vi "read_attributes.vi"(8 "error in (no error)":errorcluster, 11 "Ridge in":refnum<class "Ridge.lvclass">) -> (0 "error out":errorcluster, 2 "attributes":T1, 3 "Ridge out":refnum<class "Ridge.lvclass">)   [LabVIEW 2020, in "Ridge.lvclass"]
uses:
  Ridge.lvclass
  Controls/ridge_attributes.ctl
  Ridge.lvclass/Ridge.ctl
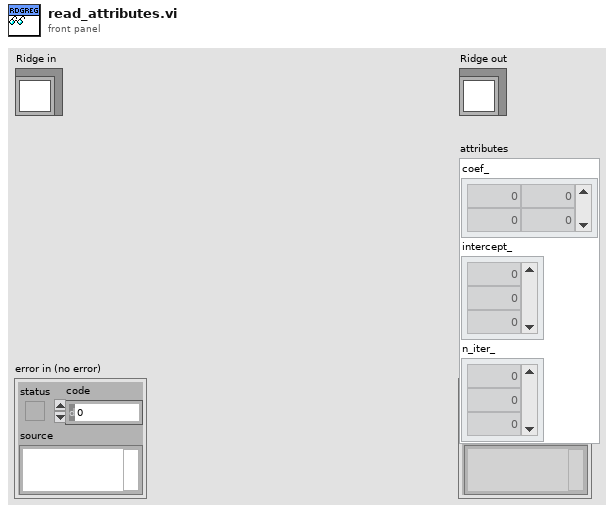
[diagram p1: front panel]
types:
  T1 = typedef "ridge_attributes.ctl" = cluster{"coef_":dbl[][], "intercept_":dbl[], "n_iter_":dbl[]}
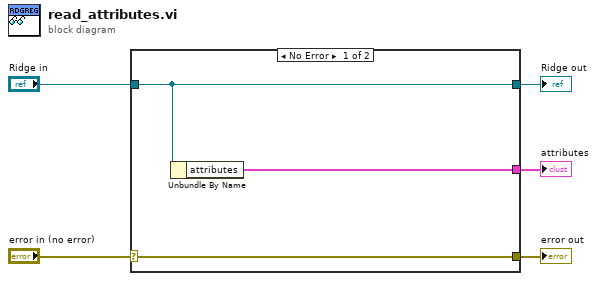
[diagram p0: block diagram]
diagram:
  n1 = case shown="No Error" "error in (no error)" {
    selector: "error in (no error)" -> [w8 w9]
    tunnel: [w8 w9] -> w4
    tunnel: [w7 w10] -> w2
    tunnel: "Ridge in" -> [w7 w10]
    tunnel: [w6 _] -> w1
    frame No Error {
      n2 = Unbundle By Name(w7) -> ("attributes"=w6:T1)
    }
    frame Error {
    }
  }
  "error out" <- w4
  "Ridge out" <- w2
  "attributes" <- w1
